vi "Write Max Amps.vi"(8 "error in (no error)":errorcluster, 10 "Max Current":dbl, 11 "PowerSupply in":refnum<class "PowerSupply.lvclass">) -> (0 "error out":errorcluster, 3 "PowerSupply out":refnum<class "PowerSupply.lvclass">)   [LabVIEW 2020, in "LAF2024Q2.lvlib" / "PowerSupply.lvclass"]
uses:
  PowerSupply.lvclass
  PowerSupply.lvclass/PowerSupply.ctl
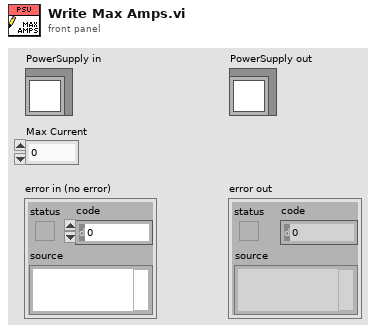
[diagram p1: front panel]
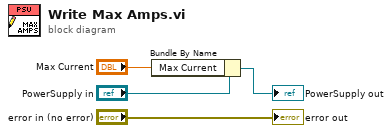
[diagram p0: block diagram]
diagram:
  n1 = Bundle By Name(cluster="PowerSupply in", "Max Current"="Max Current") -> (→"PowerSupply out":refnum<class "PowerSupply.lvclass">)
  "error out" <- "error in (no error)"
